vi "Exited.vi"(4 "User Parameter":refnum<user-event>[](array[refnum]), 5 "Event Data":cluster{"sender":refnum<k24>, "e":refnum<k24>}, 6 "Control Ref":refnum<k24>, 7 "Event Common Data":T1) -> ()   [LabVIEW 2018, in "callback-system-exec.lvlib"]
uses:
  callback-system-exec.lvlib
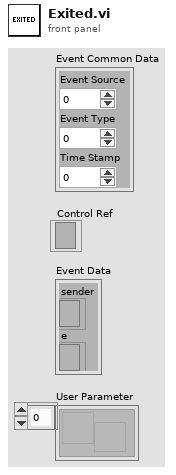
[diagram p1: front panel]
types:
  T1 = cluster{"Event Source":i32, "Event Type":u32, "Time Stamp":u32}
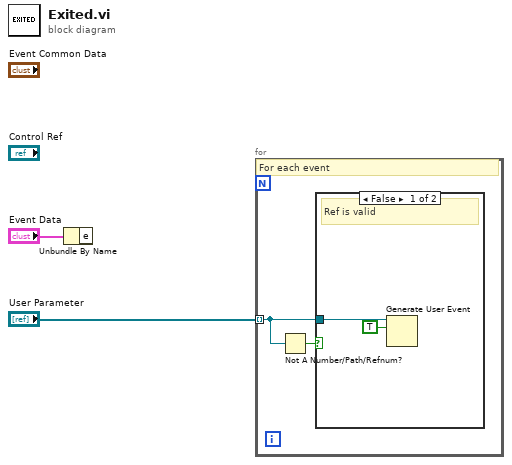
[diagram p0: block diagram]
diagram:
  n1 = Unbundle By Name("Event Data") -> ()  [unwired: 1 out]
  n2 = for {
    tunnel: "User Parameter" -> [w3] mode=indexing
    # "For each event"
    n3 = Not A Number/Path/Refnum?(number/path/refnum=w3) -> (NaN/Path/Refnum?=w4:bool)
    n4 = case shown="False" w4 {
      tunnel: w3 -> [w6 _]
      frame False {
        # "Ref is valid"
        n5 = Generate User Event(user event=w6, event data cluster=TRUE ("event data")) -> ()  [unwired: 2 in, 2 out]
      }
      frame True {
      }
    }
  }
